vi "TimeStamp_Filename.vi"() -> (0 "appended path":path)   [LabVIEW 2018]
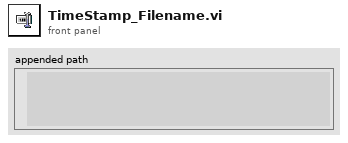
[diagram p1: front panel]
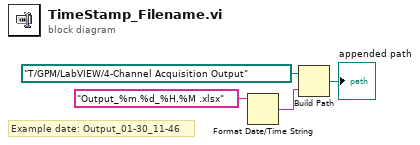
[diagram p0: block diagram]
diagram:
  # "Example date: Output_01-30_11-46"
  n1 = Format Date/Time String(time format string (%c)="Output_%m.%d_%H.%M .xlsx") -> (date/time string=w2:string)  [unwired: 2 in]
  n2 = Build Path(base path=path "T:/GPM/LabVIEW/4-Channel Acquisition Output" ("Filename"), name or relative path=w2) -> (appended path=→"appended path":path)
